vi "ep_Flicker Block1.vi"(0 "voltage waveform":waveform(dbl), 1 "init":bool, 5 "nominal frequency":enum16{"50 Hz", "60 Hz"}(ring), 7 "RMS (1/2) (half cycle)":cluster{"times":timestamp[], "RMS (1/2)":dbl[]}) -> (4 "adapted voltage":dbl[](array[numeric]))   [LabVIEW 2011, in "NI_EP_Power Quality.lvlib"]
doc: "This VI represent a voltage adapting circuit that scales the mean r.m.s. value of the input mains frequency voltage down to an internal reference level."
uses:
  <vilib>/addons/Electrical Power/PQ/NI_EP_Power Quality.lvlib
  <vilib>/Analysis/5stat.llb/RMS (DBL).vi
  <vilib>/Analysis/NI_AALPro.lvlib
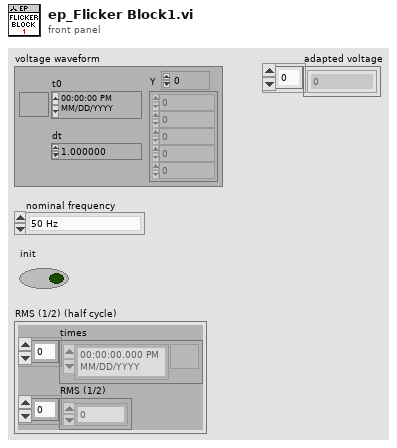
[diagram p1: front panel]
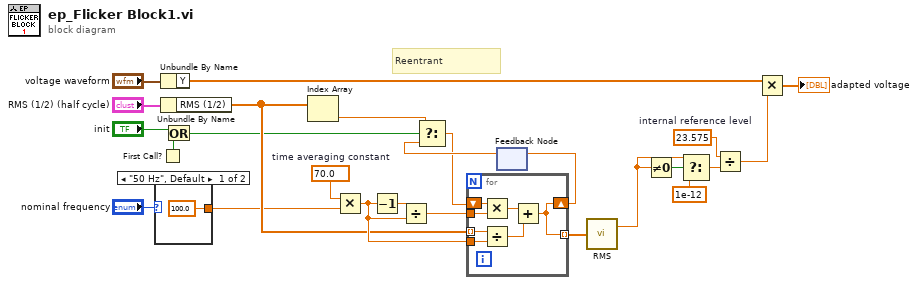
[diagram p0: block diagram]
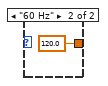
[diagram p2: hidden frame]
diagram:
  w16 = 70.0  # time averaging constant
  w9 = 23.575  # internal reference level
  # "Reentrant"
  n1 = case shown="\"50 Hz\", Default" "nominal frequency" {
    tunnel: [100.0 120.0] -> w12
    frame "50 Hz", Default {
    }
    frame "60 Hz" {
    }
  }
  n2 = First Call?() -> (First Call?: T/F=w6:bool)
  n3 = Unbundle By Name("voltage waveform") -> ("Y"=w15:dbl[])
  n4 = Unbundle By Name("RMS (1/2) (half cycle)") -> ("RMS (1/2)"=w14:dbl[])
  n5 = Or(x="init", y=w6) -> (x .or. y?=w13:bool)
  n6 = Index Array(array=w14) -> (element=w20:dbl)  [unwired: 1 in]
  n7 = Multiply(x=w16, y=w12) -> (x*y=w18:dbl)
  n8 = Decrement(x=w18) -> (x-1=w19:dbl)
  n9 = Divide(x=w19, y=w18) -> (x/y=w17:dbl)
  n10 = feedback #1() -> (w22:dbl)  [unwired: 1 in]
  n11 = Select(t=w20, s=w13, f=w22) -> (s? t:f=w21:dbl)
  n12 = for {
    tunnel: w17 -> [w33]
    tunnel: w18 -> [w32]
    shift-right: [w28] -> w23
    shift-left: w21 -> [w29]
    tunnel: w14 -> [w30] mode=indexing
    tunnel: [w28] -> w24 mode=indexing
    n13 = Multiply(x=w29, y=w33) -> (x*y=w34:dbl)
    n14 = Divide(x=w30, y=w32) -> (x/y=w31:dbl)
    n15 = Add(x=w34, y=w31) -> (x+y=w28:dbl)
  }
  n16 = feedback-in #1(w23) -> ()
  n17 = call-poly <vilib>:"RMS.vi"("X"=w24) -> ("rms value"=w25:dbl)  [unwired: 1 out]
  n18 = Not Equal To 0?(x=w25) -> (x != 0?=w2:bool)
  n19 = Select(t=w25, s=w2, f=1e-12) -> (s? t:f=w8:dbl)
  n20 = Divide(x=w9, y=w8) -> (x/y=w4:dbl)
  n21 = Multiply(x=w15, y=w4) -> (x*y=→"adapted voltage":dbl[])
